vi "TDTRX6-Init DAQ (Npts).vi"(0 "AO Fs (Hz)":dbl, 5 "AI Fs (Hz)":dbl, 7 "Num AO Pts":i32, 9 "Num AO Buffers":i32=2, 11 "error in (no error)":errorcluster, 12 "AI Channels":i32[](array[numeric])=[1, 2]) -> (4 "AO Fs (coerced)":dbl, 6 "AI Fs (coerced)":dbl, 8 "AO npts":i32, 10 "AI npts":i32, 15 "error out":errorcluster)   [LabVIEW 2015]
uses:
  TDT-Signal Bank Action.ctl
  TDT-Globals.vi
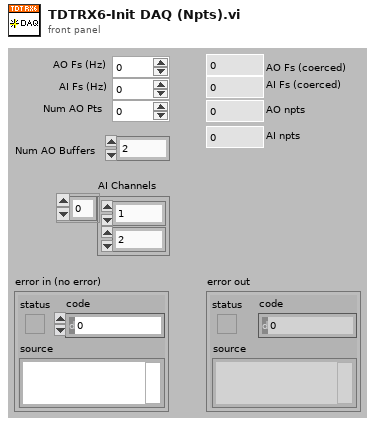
[diagram p1: front panel]
types:
  T1 = typedef "TDT-Signal Bank Action.ctl" = enum16{"Init", "Write", "Read", "Rewrite", "Reset"}
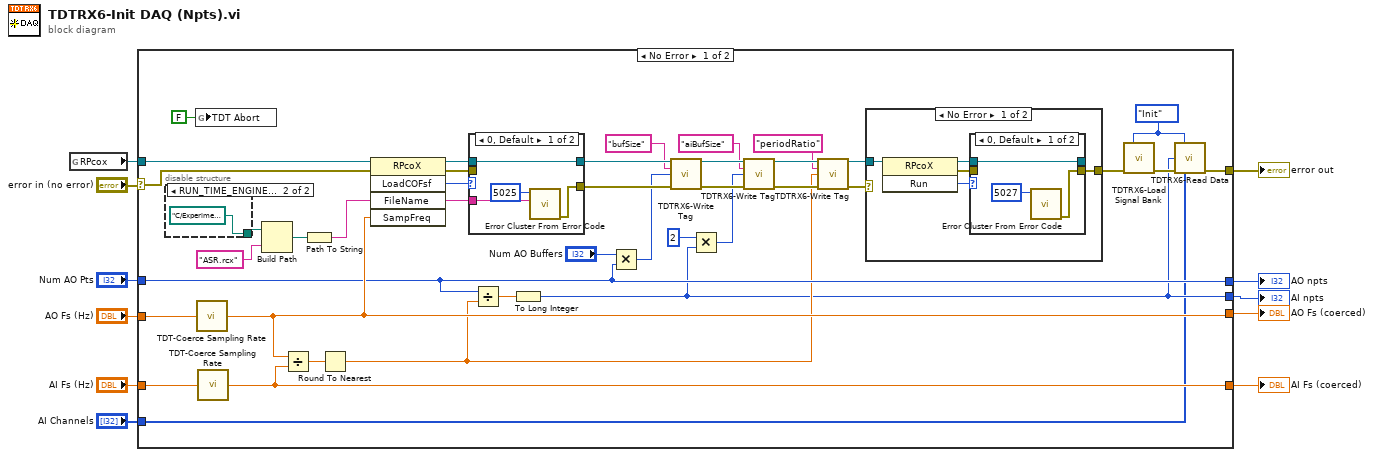
[diagram p0: block diagram]
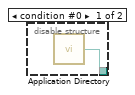
[diagram p2: hidden frame]
diagram:
  n1 = global read "TDT-Globals.vi" "RPcox"() -> (w9:refnum<k7>)
  n2 = case shown="No Error" "error in (no error)" {
    selector: "error in (no error)" -> [w49 w71]
    tunnel: [w25 w71] -> w10
    tunnel: w9 -> [w51 _]
    tunnel: "AO Fs (Hz)" -> [w29 _]
    tunnel: "AI Fs (Hz)" -> [w28 _]
    tunnel: "Num AO Pts" -> [w19 _]
    tunnel: [w27 _] -> w5
    tunnel: [w26 _] -> w4
    tunnel: [w19 _] -> w3
    tunnel: [w16 _] -> w2
    tunnel: "AI Channels" -> [w15 _]
    frame No Error {
      w24 = TDT-Signal_Bank_Action."Init" ("Action")
      n3 = disable-structure shown="RUN_TIME_ENGINE==False" {
        disable-tunnel: [w52 path "C:/Experiment VIs/PXI DAQ VIs/TDT VIs/rpfiles"] -> w13
        frame condition #0 {
          n4 = call <vilib>:"Application Directory.vi"() -> ("Application Directory"=w52:path)
        }
        frame condition #1 (active) {
        }
      }
      n5 = global write "TDT-Globals.vi" "TDT Abort"(FALSE ("TDT Abort")) -> ()
      n6 = call "TDT-Coerce Sampling Rate.vi"("Fs (Hz)"=w29) -> ("Coerced"=w27:dbl)
      n7 = call "TDT-Coerce Sampling Rate.vi"("Fs (Hz)"=w28) -> ("Coerced"=w26:dbl)
      n8 = Build Path(base path=w13, name or relative path="ASR.rcx") -> (appended path=w12:path)
      n9 = Divide(x=w27, y=w26) -> (x/y=w30:dbl)
      n10 = Path To String(path=w12) -> (string=w50:string)
      n11 = Round To Nearest(number=w30) -> (nearest integer value=w18:dbl)
      n12 = invoke class="RPcoX" method="LoadCOFsf"(reference=w51, error in=w49, "FileName"=w50, "SampFreq"=w27) -> (reference out=w46:refnum<k7>, error out=w45:errorcluster, "LoadCOFsf"=w48:i32, "FileName"=w47:string)  [unwired: 1 in, 1 out]
      n13 = case shown="0, Default" w48 {
        tunnel: w47 -> [w67 _]
        tunnel: w46 -> [w68 w70]
        tunnel: w45 -> [_ w69]
        tunnel: [w68 w70] -> w44
        tunnel: [w65 w69] -> w43
        frame 0, Default {
          n14 = call <vilib>:"Error Cluster From Error Code.vi"("error message (\"\")"=w67, "error code (0)"=5025) -> ("error out"=w65:errorcluster)  [unwired: 7 in]
        }
        frame 1 {
        }
      }
      n15 = Divide(x=w19, y=w18) -> (x/y=w17:dbl)
      n16 = To Long Integer(number=w17) -> (32bit integer=w16:i32)
      n17 = Multiply(x="Num AO Buffers", y=w19) -> (x*y=w21:i32)
      n18 = call "TDTRX6-Write Tag.vi"("RPcox"=w44, "Name"="bufSize", "Value"=w21, "error in"=w43) -> ("RPcox Out"=w40:refnum<k7>, "error out"=w41:errorcluster)  [unwired: 10 in]
      n19 = Multiply(x=2, y=w16) -> (x*y=w23:i32)
      n20 = call "TDTRX6-Write Tag.vi"("RPcox"=w40, "Name"="aiBufSize", "Value"=w23, "error in"=w41) -> ("RPcox Out"=w37:refnum<k7>, "error out"=w38:errorcluster)  [unwired: 10 in]
      n21 = call "TDTRX6-Write Tag.vi"("RPcox"=w37, "Name"="periodRatio", "Value"=w18, "error in"=w38) -> ("RPcox Out"=w35:refnum<k7>, "error out"=w33:errorcluster)  [unwired: 10 in]
      n22 = case shown="No Error" w33 {
        selector: w33 -> [_ w64]
        tunnel: w35 -> [w58 _]
        tunnel: [w55 w64] -> w34
        frame No Error {
          n23 = invoke class="RPcoX" method="Run"(reference=w58) -> (reference out=w56:refnum<k7>, error out=w57:errorcluster, "Run"=w54:i32)  [unwired: 2 in]
          n24 = case shown="0, Default" w54 {
            tunnel: w56 -> [w61 w63]
            tunnel: w57 -> [_ w62]
            tunnel: [w61 w63] -> _
            tunnel: [w59 w62] -> w55
            frame 0, Default {
              n25 = call <vilib>:"Error Cluster From Error Code.vi"("error code (0)"=5027) -> ("error out"=w59:errorcluster)  [unwired: 8 in]
            }
            frame 1 {
            }
          }
        }
        frame Error {
        }
      }
      n26 = call "TDTRX6-Load Signal Bank.vi"("Action"=w24, "error in (no error)"=w34) -> ("error out"=w32:errorcluster)  [unwired: 13 in]
      n27 = call "TDTRX6-Read Data.vi"("Action"=w24, "Pts Per Read"=w16, "error in (no error)"=w32, "AI Channels"=w15) -> ("error out"=w25:errorcluster)  [unwired: 10 in, 1 out]
    }
    frame Error {
    }
  }
  "error out" <- w10
  "AO Fs (coerced)" <- w5
  "AI Fs (coerced)" <- w4
  "AO npts" <- w3
  "AI npts" <- w2
